vi "ws_authorize summary.vi"(4 "error in (no error)":errorcluster, 6 "Authorization Request Sent? (f)":bool, 7 "Authorization":T2) -> (0 "error out":errorcluster, 3 "Template Keys":T1)   [LabVIEW 2011]
uses:
  license/Authorization Data.ctl
  <vilib>/addons/internet/utils/keyedarr.llb/Keyed Array.ctl
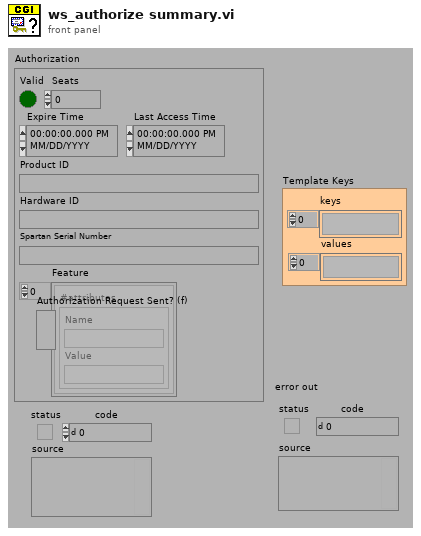
[diagram p1: front panel]
types:
  T1 = typedef "Keyed Array.ctl" = cluster{"keys":string[], "values":string[]}
  T2 = typedef "Authorization Data.ctl" = cluster{"Valid":bool, "Seats":i32, "Expire Time":timestamp, "Last Access Time":timestamp, "Product ID":string, "Hardware ID":string, "Spartan Serial Number":string, "Feature":cluster{"#attributes":cluster{"Name":string, "Value":string}}[]}
  T3 = cluster{"Days/Runs Remaining":i32, "Days/Runs Allowed":i32, "Days/Runs Used":i32}
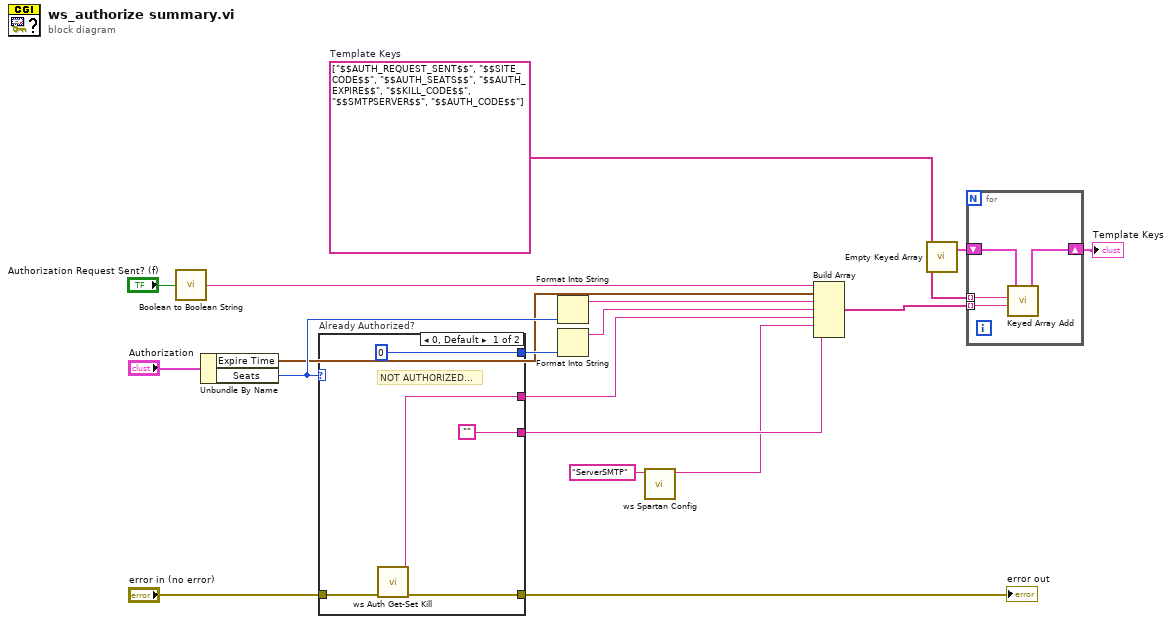
[diagram p0: block diagram]
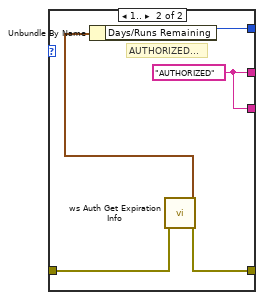
[diagram p2: hidden frame]
diagram:
  w15 = string[] ["$$AUTH_REQUEST_SENT$$", "$$SITE_CODE$$", "$$AUTH_SEATS$$", "$$AUTH_EXPIRE$$", "$$KILL_CODE$$", "$$SMTPSERVER$$", "$$AUTH_CODE$$"]  # Template Keys
  n1 = call "Boolean to Boolean String.vi"("Boolean"="Authorization Request Sent? (f)") -> ("Boolean string"=w11:string)  [unwired: 1 in]
  n2 = Unbundle By Name("Authorization") -> ("Expire Time"=w6:timestamp, "Seats"=w10:i32)
  n3 = case "Already Authorized?" shown="0, Default" w10 {
    tunnel: "error in (no error)" -> [w23 w27]
    tunnel: [w22 w26] -> w18
    tunnel: [0 ("Days/runs remaining") w24] -> w8
    tunnel: [w20 w28] -> w5
    tunnel: ["" w28] -> w3
    frame 0, Default {
      # "NOT AUTHORIZED..."
      n4 = call "ws Auth Get-Set Kill.vi"("error in (no error)"=w23) -> ("error out"=w22:errorcluster, "KillCode"=w20:string)  [unwired: 9 in]
    }
    frame 1.. {
      w28 = "AUTHORIZED"
      # "AUTHORIZED..."
      n5 = call "ws Auth Get Expiration Info.vi"("error in (no error)"=w27) -> ("error out"=w26:errorcluster, "Authorization Expiration Information"=w25:T3)  [unwired: 8 in, 1 out]
      n6 = Unbundle By Name(w25) -> ("Days/Runs Remaining"=w24:i32)
    }
  }
  "error out" <- w18
  n7 = Format Into String(w10) -> (resulting string=w9:string)  [unwired: 3 in, 1 out]
  n8 = Format Into String(w8) -> (resulting string=w7:string)  [unwired: 3 in, 1 out]
  n9 = call "ws Spartan Config.vi"("config key (\"\")"="ServerSMTP" ("config key (\"\")")) -> ("config value"=w1:string)  [unwired: 8 in, 2 out]
  n10 = Build Array(w11, w6, w9, w7, w5, w1, w3) -> (w14:string[])
  n11 = call "Empty Keyed Array.vi"() -> ("empty keyed array"=w13:T1)  [unwired: 3 out]
  n12 = for {
    tunnel: w15 -> [w32] mode=indexing
    tunnel: w14 -> [w31] mode=indexing
    shift-right: [w30] -> w12
    shift-left: w13 -> [w29]
    n13 = call <vilib>:"Keyed Array Add.vi"("value"=w31, "key"=w32, "array in"=w29) -> ("array out"=w30:T1)  [unwired: 1 in, 3 out]
  }
  "Template Keys" <- w12
